vi "Index Global.vi"() -> ()   [LabVIEW 2019]
panel:
  in  "Index Motor Values":dbl
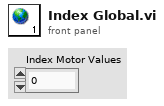
[diagram p1: front panel]
diagram:
